vi "Write Data.vi"(8 "error in (no error)":errorcluster, 9 "Publication Time":timestamp, 10 "Value":variant, 11 "ListboxItemNamesBinding In":refnum<class "ListboxItemNamesBinding.lvclass">) -> (0 "error out":errorcluster, 3 "ListboxItemNamesBinding Out":refnum<class "ListboxItemNamesBinding.lvclass">)   [LabVIEW 2020, in "ListboxItemNamesBinding.lvclass"]
doc: "<License>\nCopyright © 2017 Composed Systems, LLC | All rights reserved\nwww.composed.io\n\nAuthor: Ethan Stern <ethan.stern@composed.io>\n\nThis software is provided \"AS IS\" WITHOUT WARRANTIES, either express or implied, AND IS FOR EDUCATIONAL PURPOSES ONLY.\n</License>"
uses:
  <vilib>/gpm_packages/@cs/transport/Source/Concrete/ListboxItemNamesBinding/ListboxItemNamesBinding.lvclass
  <vilib>/gpm_packages/@cs/transport/Source/Concrete/ListboxItemNamesBinding/ListboxItemNamesBinding.lvclass/ListboxItemNamesBinding.ctl
  <vilib>/Utility/error.llb/Error Cluster From Error Code.vi
  <vilib>/ErrorRing/Error Ring.xnode
  <vilib>/Utility/Data Type/NI_Data Type.lvlib
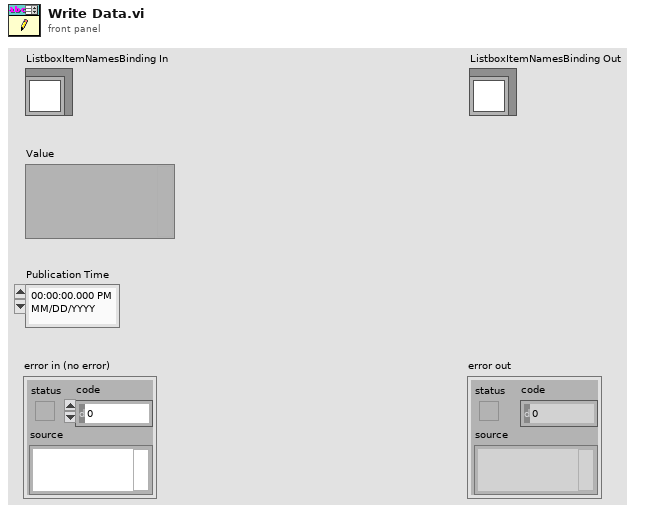
[diagram p1: front panel]
types:
  T1 = typedef "ListboxItemNamesBinding.lvclass/Listbox Binding Options.ctl" = bool
  T2 = typedef "NI_Data Type.lvlib/Data Type.ctl" = enum8{"Invalid Type", "Void", "I8", "I16", "I32", "I64", "U8", "U16", "U32", "U64", "Single Float", "Double Float", "Extended Float", "Single Complex", "Double Complex", "Extended Complex", "Enum U8", "Enum U16", "Enum U32", "Enum U64", "Single Float With Unit", "Double Float With Unit", "Extended Float With Unit", "Single Complex with Unit", "Double Complex with Unit", "Extended Complex with Unit", "Boolean", "String", "Path", "Picture", "Tag", "Array", "Cluster", "Variant", "LV Variant", "Waveform", "Timestamp", "Digital Waveform", "Digital Data", "ExpressData", "Refnum", "External Data", "VI", "Poly VI", "LabVIEW Class Instance", "Fixed Point", "Set Collection", "Map Collection"}
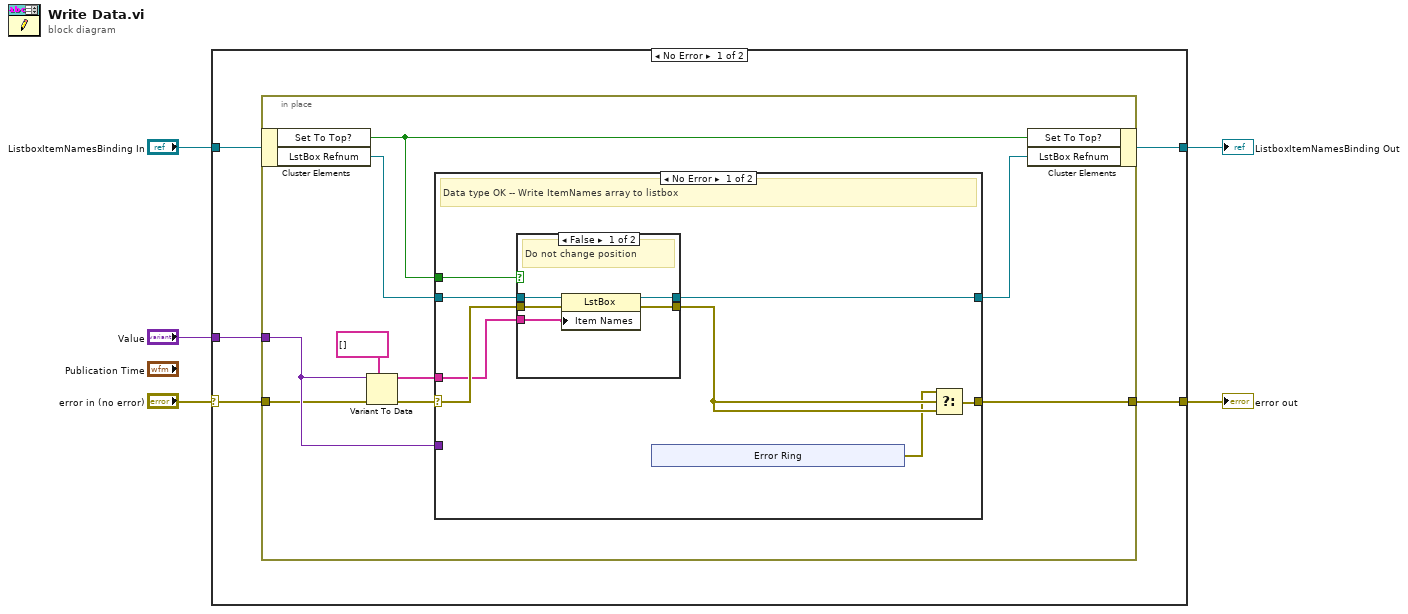
[diagram p0: block diagram]
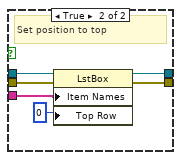
[diagram p2: hidden frame]
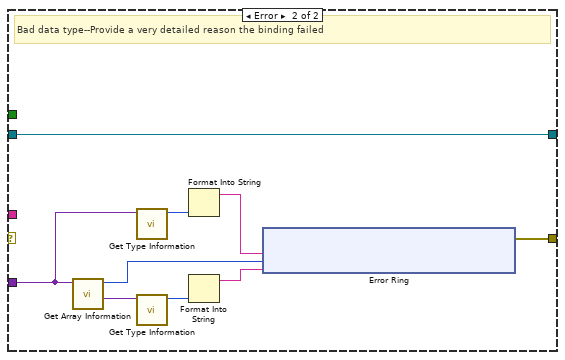
[diagram p3: hidden frame]
diagram:
  n1 = case shown="No Error" "error in (no error)" {
    selector: "error in (no error)" -> [w6 w62]
    tunnel: "Value" -> [w10 _]
    tunnel: [w9 w62] -> w4
    tunnel: "ListboxItemNamesBinding In" -> [w8 w63]
    tunnel: [w7 w63] -> w2
    frame No Error {
      n2 = in-place {
        in-place-border: w10 -> [w19]
        in-place-border: [w15] -> w9
        in-place-border: w6 -> [w12]
        n3 = in-place-cluster #1(w8) -> ("Set To Top?"=w11:T1, "LstBox Refnum"=w14:refnum<vi>)
        n4 = Variant To Data(error in=w12, type=string[] [], Variant=w19) -> (data=w16:string[], error out=w17:errorcluster)
        n5 = case shown="No Error" w17 {
          selector: w17 -> [w26 _]
          tunnel: w16 -> [w25 _]
          tunnel: w14 -> [w27 w50]
          tunnel: w19 -> [_ w51]
          tunnel: w11 -> [w24 _]
          tunnel: [w22 w52] -> w15
          tunnel: [w23 w50] -> w13
          frame No Error {
            # "Data type OK -- Write ItemNames array to listbox"
            n6 = case shown="False" w24 {
              tunnel: w27 -> [w37 w43]
              tunnel: w26 -> [w36 w42]
              tunnel: w25 -> [w34 w41]
              tunnel: [w35 w40] -> w21
              tunnel: [w33 w38] -> w23
              frame False {
                # "Do not change position"
                n7 = property class="LstBox"(reference=w37, error in=w36, "Item Names"=w34) -> (reference out=w33:refnum<vi>, error out=w35:errorcluster)
              }
              frame True {
                # "Set position to top"
                n8 = property class="LstBox"(reference=w43, error in=w42, "Item Names"=w41, "Top Row"=0) -> (reference out=w38:refnum<vi>, error out=w40:errorcluster)
              }
            }
            n9 = xnode "Error Ring"() -> ("error out"=w20:errorcluster)
            n10 = Select(t=w20, s=w21, f=w21) -> (s? t:f=w22:errorcluster)
          }
          frame Error {
            # "Bad data type--Provide a very detailed reason the binding failed"
            n11 = call <vilib>:"Get Array Information.vi"("variant"=w51) -> ("array element data type"=w49:variant, "number of dimensions"=w45:i32)  [unwired: 7 in, 2 out]
            n12 = call <vilib>:"Get Type Information.vi"("variant"=w51) -> ("type"=w47:T2)  [unwired: 6 in, 4 out]
            n13 = call <vilib>:"Get Type Information.vi"("variant"=w49) -> ("type"=w48:T2)  [unwired: 6 in, 4 out]
            n14 = Format Into String(w47) -> (resulting string=w46:string)  [unwired: 3 in, 1 out]
            n15 = Format Into String(w48) -> (resulting string=w44:string)  [unwired: 3 in, 1 out]
            n16 = xnode "Error Ring"("parameter 0"=w46, "parameter 1"=w45, "parameter 2"=w44) -> ("error out"=w52:errorcluster)
          }
        }
        n17 = in-place-cluster #1("Set To Top?"=w11, "LstBox Refnum"=w13) -> (w7:refnum<class "ListboxItemNamesBinding.lvclass">)
      }
    }
    frame Error {
    }
  }
  "error out" <- w4
  "ListboxItemNamesBinding Out" <- w2
